vi "快关终端速度.vi"(3 "计算参数 in":T1, 4 "Sampling Rate":dbl, 5 "Array in":dbl[](array[numeric])) -> (0 "计算参数 out":T1, 2 "Array out":dbl[](array[numeric]))   [LabVIEW 2013]
doc: "快关试验的终端速度存放在DFT中。"
uses:
  <vilib>/Analysis/NI_AALPro.lvlib
panel:
  out "EV":dbl
  out "Y":dbl[](array[numeric])
  out "X":dbl[](array[numeric])
  out "start":dbl
  out "step":dbl
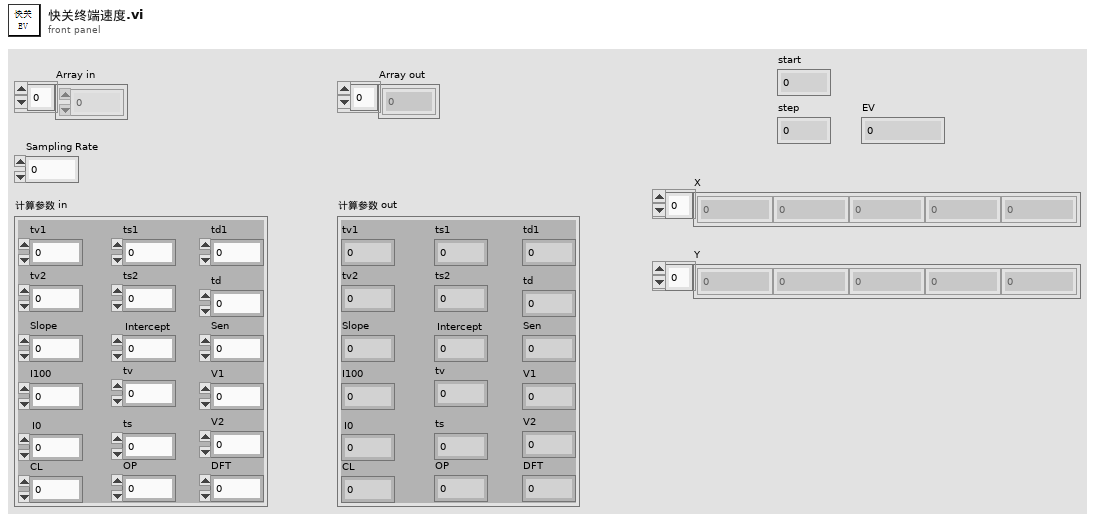
[diagram p1: front panel]
types:
  T1 = cluster{"tv1":dbl, "tv2":dbl, "tv":dbl, "ts1":dbl, "ts2":dbl, "ts":dbl, "td1":dbl, "td":dbl, "Slope":dbl, "Intercept":dbl, "I100":dbl, "I0":dbl, "Sen":dbl, "V1":dbl, "V2":dbl, "CL":dbl, "OP":dbl, "DFT":dbl}
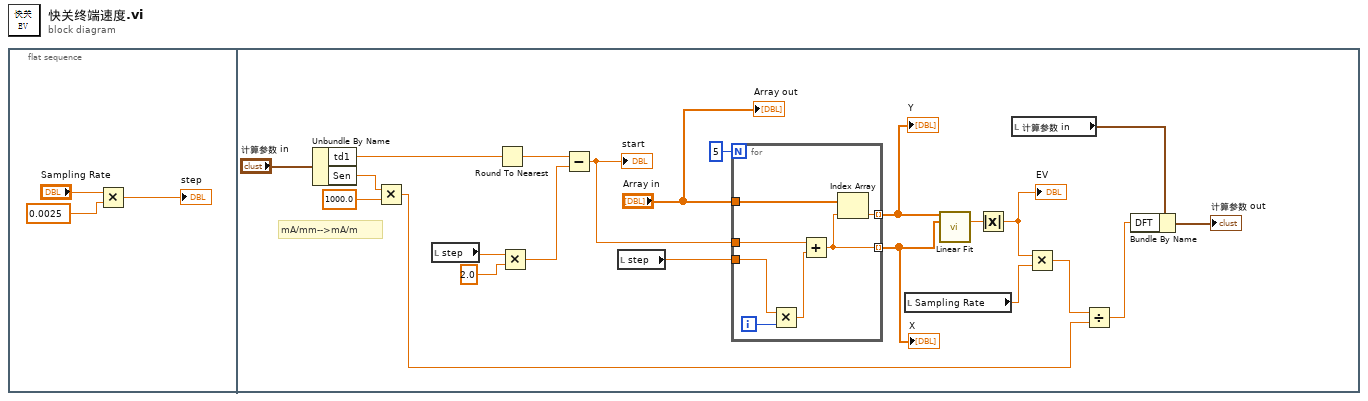
[diagram p0: block diagram]
diagram:
  n1 = flat-sequence {
    frame #0 {
      n2 = Multiply(x="Sampling Rate", y=0.0025) -> (x*y=→"step":dbl)
    }
    frame #1 {
      # "mA/mm-->mA/m"
      n3 = Unbundle By Name("计算参数 in") -> ("td1"=w24:dbl, "Sen"=w6:dbl)
      n4 = Multiply(x=w6, y=1000.0) -> (x*y=w4:dbl)
      n5 = local read "step"() -> (w22:dbl)
      n6 = Round To Nearest(number=w24) -> (nearest integer value=w25:dbl)
      n7 = Multiply(x=w22, y=2.0) -> (x*y=w19:dbl)
      n8 = Subtract(x=w25, y=w19) -> (x-y=w18:dbl)
      "start" <- w18
      n9 = local read "step"() -> (w8:dbl)
      n10 = for {
        N: 5 -> [_]
        tunnel: w8 -> [w31]
        tunnel: w18 -> [w29]
        tunnel: [w27] -> w17 mode=indexing
        tunnel: "Array in" -> [w28]
        tunnel: [w26] -> w16 mode=indexing
        i -> [w32]
        n11 = Multiply(x=w31, y=w32) -> (x*y=w30:dbl)
        n12 = Add(x=w29, y=w30) -> (x+y=w27:dbl)
        n13 = Index Array(array=w28, index=w27) -> (element=w26:dbl)
      }
      "Y" <- w16
      "X" <- w17
      n14 = local read "Sampling Rate"() -> (w11:dbl)
      n15 = call <vilib>:"Linear Fit.vi"("Y"=w16, "X"=w17) -> ("slope"=w12:dbl)  [unwired: 9 in, 4 out]
      n16 = Absolute Value(x=w12) -> (abs(x)=w7:dbl)
      "EV" <- w7
      n17 = local read "计算参数 in"() -> (w15:T1)
      n18 = Multiply(x=w7, y=w11) -> (x*y=w10:dbl)
      n19 = Divide(x=w10, y=w4) -> (x/y=w9:dbl)
      n20 = Bundle By Name(cluster=w15, "DFT"=w9) -> (→"计算参数 out":T1)
      "Array out" <- "Array in"
    }
  }
